vi "MusicPlayer_Create.vi"(0 "reference in":refnum<class "MusicPlayer.lvclass">, 11 "Error In":errorcluster) -> (4 "reference out":refnum<class "MusicPlayer.lvclass">, 15 "Error Out":errorcluster)   [LabVIEW 2022 SP3, in "MusicPlayer.lvclass"]
uses:
  MusicPlayer.lvclass
  MusicPlayer.lvclass/MusicPlayer.ctl
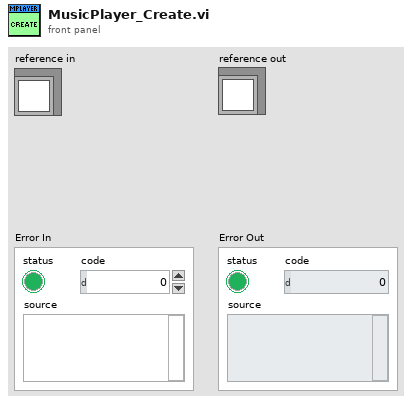
[diagram p1: front panel]
types:
  T1 = typedef "MusicPlayer.lvclass/ObjectAttributes.ctl" = cluster{"MediaPlayer":refnum<k7>}
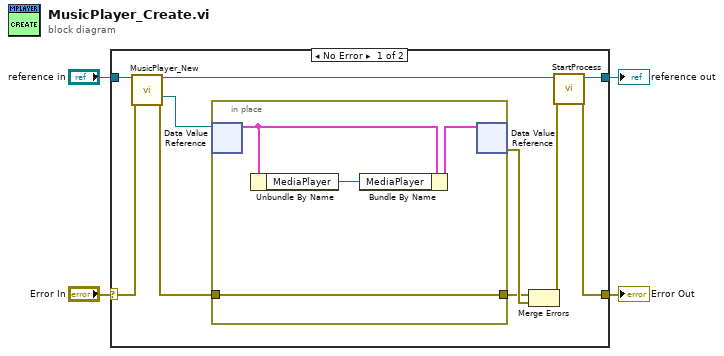
[diagram p0: block diagram]
diagram:
  n1 = case shown="No Error" "Error In" {
    selector: "Error In" -> [w13 w20]
    tunnel: [w5 w20] -> w3
    tunnel: "reference in" -> [w14 w19]
    tunnel: [w7 w19] -> w1
    frame No Error {
      n2 = call "MusicPlayer_New.vi"("reference in"=w14, "error in (no error)"=w13) -> ("reference out"=w8:refnum<class "MusicPlayer.lvclass">, "DVRRefOut"=w11:refnum<data-value>, "error out"=w10:errorcluster)  [unwired: 10 in, 1 out]
      n3 = in-place {
        in-place-border: w10 -> [w15]
        in-place-border: [w15] -> w9
        n4 = in-place-dvr #1(w11) -> (w17:T1)  [unwired: 1 out]
        n5 = Unbundle By Name(w17) -> ("MediaPlayer"=w16:refnum<k7>)
        n6 = Bundle By Name(cluster=w17, "MediaPlayer"=w16) -> (w18:T1)
        n7 = in-place-dvr #1(w18) -> (w12:errorcluster)  [unwired: 1 out]
      }
      n8 = Merge Errors(w9, w12) -> (w6:errorcluster)
      n9 = call "StartProcess.vi"("reference in"=w8, "Error In"=w6) -> ("reference out"=w7:refnum<class "MusicPlayer.lvclass">, "Error Out"=w5:errorcluster)  [unwired: 14 in, 2 out]
    }
    frame Error {
      # "VI-TechBaseTemplate_Simple_4x4x4"
    }
  }
  "Error Out" <- w3
  "reference out" <- w1
